vi "delete cero.vi"(11 "Array in":dbl[](array[numeric])) -> (3 "Array 3":dbl[](array[numeric]))   [LabVIEW 2012]
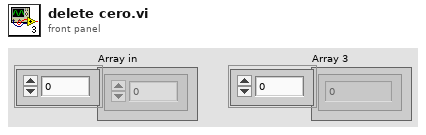
[diagram p1: front panel]
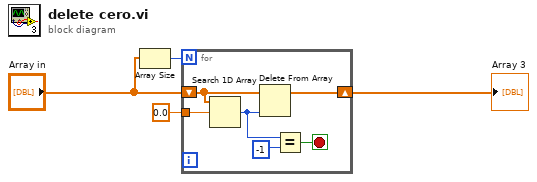
[diagram p0: block diagram]
diagram:
  n1 = Array Size(array="Array in") -> (size(s)=w2:i32)
  n2 = for {
    N: w2 -> [_]
    shift-right: [w9] -> w3
    shift-left: "Array in" -> [w10]
    tunnel: 0.0 ("element") -> [w8]
    stop <- w5 stop-if-true
    n3 = Search 1D Array(1D array=w10, element=w8) -> (index of element=w7:i32)  [unwired: 1 in]
    n4 = Delete From Array(array=w10, index=w7) -> (array with subset deleted=w9:dbl[])  [unwired: 1 in, 1 out]
    n5 = Equal?(x=w7, y=-1) -> (x = y?=w5:bool)
  }
  "Array 3" <- w3
